vi "Choreo_ReadAllTrajectoryFile_Example.vi"() -> (0 "error out":errorcluster)   [LabVIEW 2019]
uses:
  <vilib>/Rock Robotics/WPI/ThirdParty/ChoreoLib/ChoreoLib.lvlib
panel:
  out "Trajectory List":string[](array[string])
  in  "Read All File":bool
  # "THIS EXAMPLE READS ALL TRAJECTORIES INTO THE CACHE"
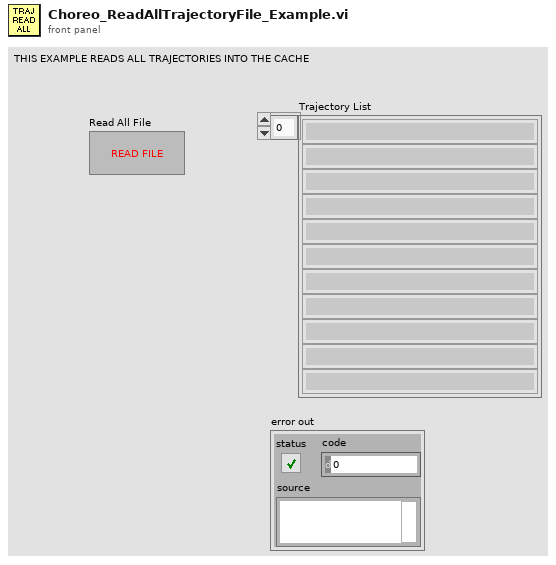
[diagram p1: front panel]
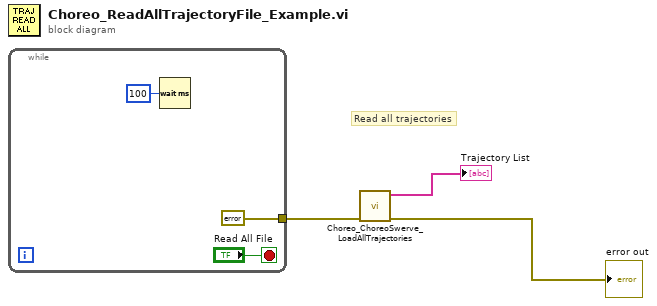
[diagram p0: block diagram]
diagram:
  # "Read all trajectories"
  n1 = while {
    tunnel: [errorcluster {"status"=FALSE, "code"=0, "source"=""} ("error in (no error)")] -> w3
    stop <- "Read All File" stop-if-true
    n2 = Wait (ms)(milliseconds to wait=u32 100) -> ()  [unwired: 1 out]
  }
  n3 = call <vilib>:"Choreo_ChoreoSwerve_LoadAllTrajectories.vi"("error in (no error)"=w3) -> ("error out"=→"error out":errorcluster, "Trajectories"=→"Trajectory List":string[])  [unwired: 9 in]
